vi "Detect Frequenza & Numero Punti Frame.vi"(9 "Np_Analysis":i32, 10 "fc - Sampling frequency \nof the card":dbl, 11 "Signal":dbl[](array[numeric])) -> (1 "Npp_Frame":i32, 3 "fs - Detected frequency \nof the signal":dbl format="%.2p")   [LabVIEW 2018]
uses:
  <vilib>/measure/NI_MAPro.lvlib
  <vilib>/measure/matone.llb/Extract Single Tone Information 1 Chan.vi
panel:
  out "Signal Waveform":waveform(dbl)(graph)
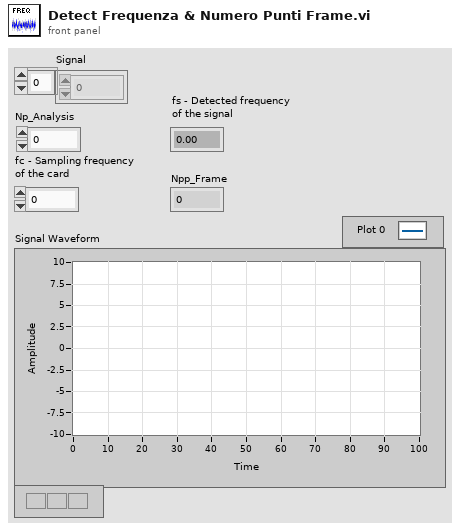
[diagram p1: front panel]
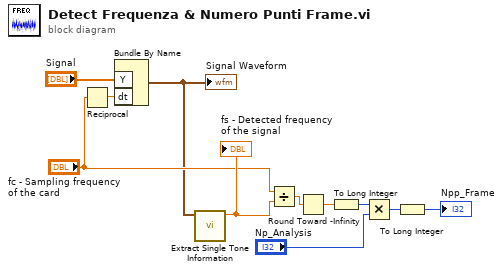
[diagram p0: block diagram]
diagram:
  n1 = Reciprocal(x="fc - Sampling frequency \nof the card") -> (1/x=w3:dbl)
  n2 = Bundle By Name("Y"="Signal", "dt"=w3) -> (w1:waveform(dbl))  [unwired: 1 in]
  "Signal Waveform" <- w1
  n3 = call-poly <vilib>:"Extract Single Tone Information.vi"("time signal in"=w1) -> ("detected frequency"=w8:dbl)  [unwired: 5 in, 5 out]
  "fs - Detected frequency \nof the signal" <- w8
  n4 = Divide(x="fc - Sampling frequency \nof the card", y=w8) -> (x/y=w9:dbl)
  n5 = Round Toward -Infinity(1:w9) -> (0:w5:dbl)
  n6 = To Long Integer(number=w5) -> (32bit integer=w4:i32)
  n7 = Multiply(x=w4, y="Np_Analysis") -> (x*y=w10:i32)
  n8 = To Long Integer(number=w10) -> (32bit integer=→"Npp_Frame":i32)
